vi "track_particle_2d.vi"(4 "Output to Image":bool=TRUE, 5 "margin":i32=15, 6 "Method":T2(ring), 7 "Optional Rectangle":i32[](array[numeric]), 9 "Threshold":sgl(slide)=128.0 scale=0.0..255.0, 11 "Image Src":T1) -> (1 "Debug Cluster":T3, 2 "Particle Position":cluster{dbl, dbl}, 3 "Image Out":T1)   [LabVIEW 2010]
uses:
  <vilib>/vision/Image Controls.llb/IMAQ Image.ctl
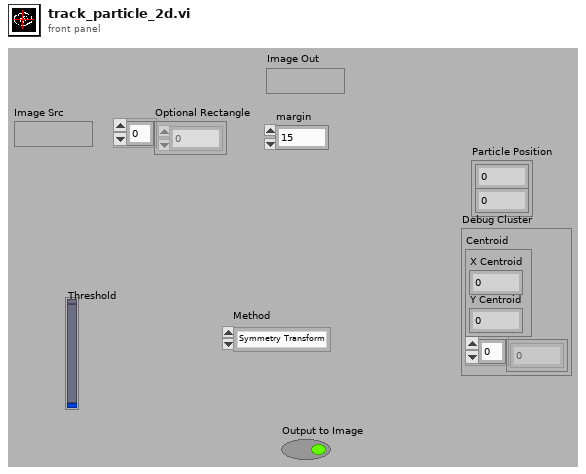
[diagram p1: front panel]
types:
  T1 = typedef "IMAQ Image.ctl" = refnum<image>
  T2 = enum16{"Symmetry Transform", "Centre of Mass", "CoM plus line information", "Inverted CoM"}
  T3 = cluster{"Centroid":cluster{"X Centroid":sgl, "Y Centroid":sgl}, i32[]}
  T4 = cluster{"Optional Rectangle[0]":i32, "Optional Rectangle[1]":i32}
  T5 = cluster{"Centroid":cluster{"X Centroid":sgl, "Y Centroid":sgl}, "Optional Rectangle":i32[]}
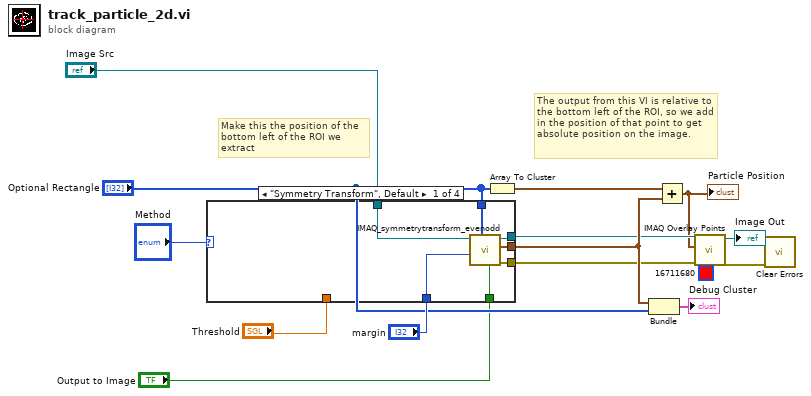
[diagram p0: block diagram]
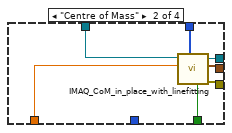
[diagram p2: hidden frame]
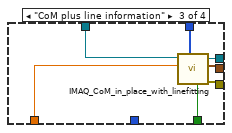
[diagram p3: hidden frame]
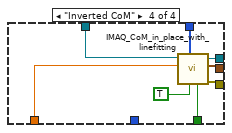
[diagram p4: hidden frame]
diagram:
  # "The output from this VI is relative to the bottom left of the ROI, so we add in the position of that point to get absolute position on the image."
  # "Make this the position of the bottom left of the ROI we extract"
  n1 = case shown="\"Symmetry Transform\", Default" "Method" {
    tunnel: "Image Src" -> [w22 w29 w36 w44]
    tunnel: [w21 w24 w31 w39] -> w4
    tunnel: [w20 w25 w32 w40] -> w14
    tunnel: "Optional Rectangle" -> [w19 w27 w34 w42]
    tunnel: "margin" -> [w18 _ _ _]
    tunnel: "Output to Image" -> [w17 w28 w35 w43]
    tunnel: "Threshold" -> [_ w26 w33 w41]
    tunnel: [w16 w23 w30 w38] -> w5
    frame "Symmetry Transform", Default {
      n2 = call "IMAQ_symmetrytransform_evenodd.vi"("Destructive"=w17, "Optional Rectangle"=w19, "margin"=w18, "Image Src"=w22) -> ("error out"=w21:errorcluster, "Centroid"=w20:cluster{"X Centroid":sgl, "Y Centroid":sgl}, "Image Src Dup"=w16:T1)  [unwired: 3 in]
    }
    frame "Centre of Mass" {
      n3 = call "IMAQ_CoM_in_place_with_linefitting.vi"("Destructive"=w28, "Optional Rectangle"=w27, "background"=w26, "Image Src"=w29) -> ("error out"=w24:errorcluster, "Centroid"=w25:cluster{"X Centroid":sgl, "Y Centroid":sgl}, "Image Src Dup"=w23:T1)  [unwired: 4 in, 1 out]
    }
    frame "CoM plus line information" {
      n4 = call "IMAQ_CoM_in_place_with_linefitting.vi"("Destructive"=w35, "Optional Rectangle"=w34, "background"=w33, "Image Src"=w36) -> ("error out"=w31:errorcluster, "Centroid"=w32:cluster{"X Centroid":sgl, "Y Centroid":sgl}, "Image Src Dup"=w30:T1)  [unwired: 4 in, 1 out]
    }
    frame "Inverted CoM" {
      n5 = call "IMAQ_CoM_in_place_with_linefitting.vi"("Destructive"=w43, "Inverted"=TRUE, "Optional Rectangle"=w42, "background"=w41, "Image Src"=w44) -> ("error out"=w39:errorcluster, "Centroid"=w40:cluster{"X Centroid":sgl, "Y Centroid":sgl}, "Image Src Dup"=w38:T1)  [unwired: 3 in, 1 out]
    }
  }
  n6 = Array To Cluster(array="Optional Rectangle") -> (cluster=w10:T4)
  n7 = Bundle("Centroid"=w14, "Optional Rectangle"="Optional Rectangle") -> (→"Debug Cluster":T5)  [unwired: 1 out]
  n8 = Add(x=w10, y=w14) -> (x+y=w2:cluster{sgl, sgl})
  "Particle Position" <- w2
  n9 = call "IMAQ Overlay Points"("Color"=u32 16711680, "error in (no error)"=w4, "Point"=w2, "Image"=w5) -> ("error out"=w1:errorcluster, "Image Out"=→"Image Out":T1)  [unwired: 6 in]
  n10 = call <vilib>:"Clear Errors.vi"("error in (no error)"=w1) -> ()  [unwired: 7 out]
